vi "Build_Version.vi"() -> (0 "Version":string)   [LabVIEW 2020]
uses:
  <vilib>/AppBuilder/AB_API_Simple/Get Build Specification Version (path).vi
  <vilib>/AppBuilder/AB_API_Simple/NI_App_Builder_API.lvlib
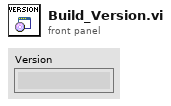
[diagram p1: front panel]
types:
  T1 = enum32{"invalid app kind", "Development System", "Run Time System", "Student Edition", "Embedded LabVIEW", "Evaluation", "Custom"}
  T2 = typedef "NI_App_Builder_API.lvlib/Build Specification Version.ctl" = cluster{"Major":u16, "Minor":u16, "Fix":u16, "Build":u16}
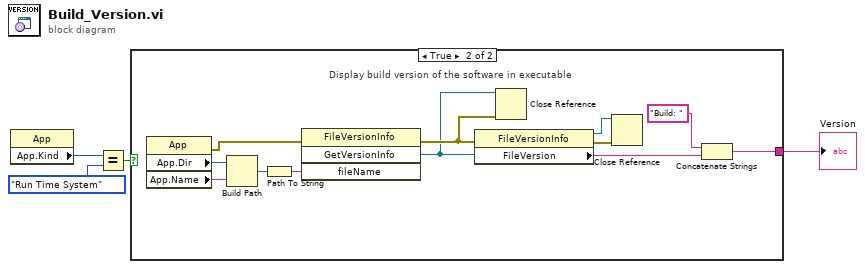
[diagram p0: block diagram]
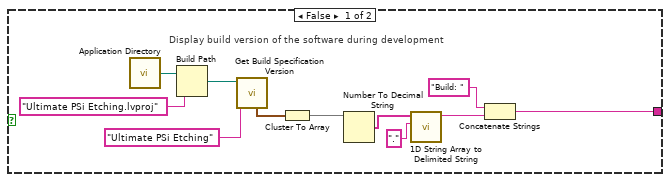
[diagram p2: hidden frame]
diagram:
  n1 = property class="App"() -> ("App.Kind"=w3:T1)  [unwired: 2 in, 2 out]
  n2 = Equal?(x=w3, y=T1."Run Time System") -> (x = y?=w4:bool)
  n3 = case shown="True" w4 {
    tunnel: [w6 w17] -> w1
    frame False {
      # "Display build version of the software during development"
      n4 = call <vilib>:"Application Directory.vi"() -> ("Application Directory"=w13:path)
      n5 = Build Path(base path=w13, name or relative path="Ultimate PSi Etching.lvproj") -> (appended path=w15:path)
      n6 = call-poly <vilib>:"Get Build Specification Version.vi"("Name of build specification"="Ultimate PSi Etching", "Path to project"=w15) -> ("Build Specification Version"=w11:T2)  [unwired: 8 in, 1 out]
      n7 = Cluster To Array(cluster=w11) -> (array=w10:u16[])
      n8 = Number To Decimal String(number=w10) -> (decimal integer string=w9:string[])  [unwired: 1 in]
      n9 = call <vilib>:"1D String Array to Delimited String.vi"("delimiter"=".", "string array"=w9) -> ("delimited string"=w7:string)  [unwired: 9 in]
      n10 = Concatenate Strings("Build: " ("string"), w7) -> (w6:string)
    }
    frame True {
      # "Display build version of the software in executable"
      n11 = property class="App"() -> (error out=w22:errorcluster, "App.Dir"=w27:path, "App.Name"=w26:string)  [unwired: 2 in, 1 out]
      n12 = Build Path(base path=w27, name or relative path=w26) -> (appended path=w25:path)
      n13 = Path To String(path=w25) -> (string=w24:string)
      n14 = invoke class="FileVersionInfo" method="GetVersionInfo"(error in=w22, "fileName"=w24) -> (error out=w20:errorcluster, "GetVersionInfo"=w19:refnum<k24>)  [unwired: 2 in, 2 out]
      n15 = property class="FileVersionInfo"(reference=w19, error in=w20) -> (reference out=w23:refnum<k24>, error out=w21:errorcluster, "FileVersion"=w18:string)
      n16 = Close Reference(reference=w19, error in (no error)=w20) -> ()  [unwired: 1 out]
      n17 = Close Reference(reference=w23, error in (no error)=w21) -> ()  [unwired: 1 out]
      n18 = Concatenate Strings("Build: " ("string"), w18) -> (w17:string)
    }
  }
  "Version" <- w1
